vi "mod_Generate Sync Parameters.vi"   [LabVIEW 2020, in "niDMT.lvlib"]
doc: "WARNING DEPRECATED DO NOT CALL FROM NEW CODE"
uses:
  <vilib>/addons/Modulation/niDMT.lvlib
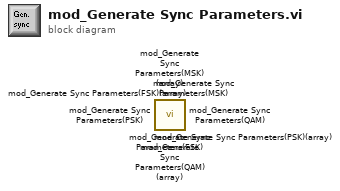
[diagram p0: block diagram]
diagram:
  n1 = call <vilib>:"mod_Generate Sync Parameters(FSK).vi"() -> ()  [unwired: 14 in, 2 out]
  n2 = call <vilib>:"mod_Generate Sync Parameters(MSK).vi"() -> ()  [unwired: 14 in, 2 out]
  n3 = call <vilib>:"mod_Generate Sync Parameters(PSK).vi"() -> ()  [unwired: 14 in, 2 out]
  n4 = call <vilib>:"mod_Generate Sync Parameters(QAM).vi"() -> ()  [unwired: 14 in, 2 out]
  n5 = call <vilib>:"mod_Generate Sync Parameters(FSK)(array).vi"() -> ()  [unwired: 14 in, 2 out]
  n6 = call <vilib>:"mod_Generate Sync Parameters(MSK)(array).vi"() -> ()  [unwired: 14 in, 2 out]
  n7 = call <vilib>:"mod_Generate Sync Parameters(PSK)(array).vi"() -> ()  [unwired: 14 in, 2 out]
  n8 = call <vilib>:"mod_Generate Sync Parameters(QAM)(array).vi"() -> ()  [unwired: 14 in, 2 out]
